vi "IFile Open.vi"(8 "error in (no error)":errorcluster, 11 "INIScoreFile in":refnum<class "INIScoreFile.lvclass">) -> (0 "error out":errorcluster, 3 "INIScoreFile out":refnum<class "INIScoreFile.lvclass">)   [LabVIEW 2020, in "INIScoreFile.lvclass"]
uses:
  INIScoreFile.lvclass
  INIScoreFile.lvclass/INIScoreFile.ctl
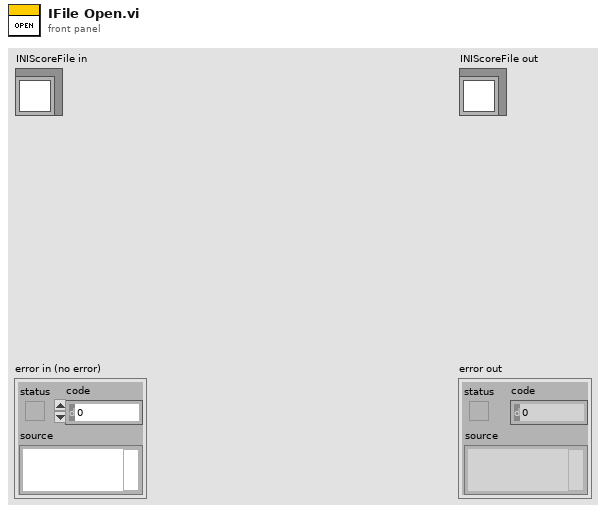
[diagram p1: front panel]
types:
  T1 = enum16{"open", "replace", "create", "open or create", "replace or create", "replace or create with confirmation"}
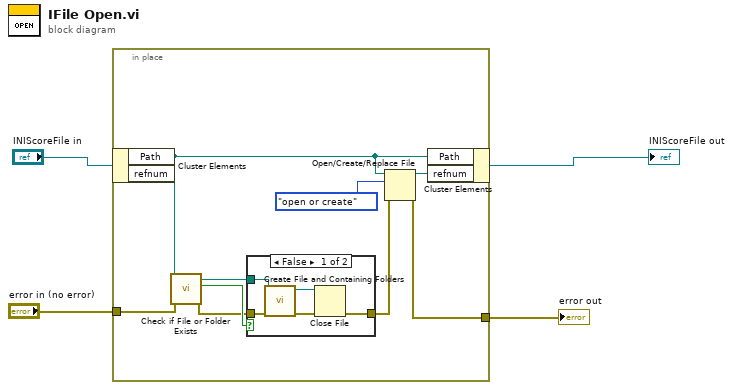
[diagram p0: block diagram]
diagram:
  n1 = in-place {
    in-place-border: "error in (no error)" -> [w8]
    in-place-border: [w12] -> w1
    n2 = in-place-cluster #1("INIScoreFile in") -> ("Path"=w10:path)  [unwired: 1 out]
    n3 = call <vilib>:"Check if File or Folder Exists.vi"("error in (no error)"=w8, "path"=w10) -> ("error out"=w7:errorcluster, "file or folder exists?"=w9:bool, "dup path"=w5:path)  [unwired: 7 in]
    n4 = case shown="False" w9 {
      tunnel: w7 -> [w18 w19]
      tunnel: [w14 w19] -> w6
      tunnel: w5 -> [w17 _]
      frame False {
        n5 = call <vilib>:"Create File and Containing Folders.vi"("error in (no error)"=w18, "file path"=w17) -> ("error out"=w16:errorcluster, "refnum out"=w15:refnum<file>)  [unwired: 8 in]
        n6 = Close File(refnum=w15, error in=w16) -> (error out=w14:errorcluster)  [unwired: 1 out]
      }
      frame True {
      }
    }
    n7 = Open/Create/Replace File(file path (use dialog)=w10, error in=w6, operation (0:open)=T1."open or create") -> (refnum out=w13:refnum<file>, error out=w12:errorcluster)  [unwired: 3 in, 1 out]
    n8 = in-place-cluster #1("Path"=w10, "refnum"=w13) -> (→"INIScoreFile out":refnum<class "INIScoreFile.lvclass">)
  }
  "error out" <- w1
